vi "Msg.Event.Fire.vi"(8 "Error (in)":errorcluster, 9 "Data":variant, 10 "Message":string, 11 "Msg.Event.Ref":T1) -> (0 "Error (out)":errorcluster, 3 "Msg.Event.Ref (out)":T1)   [LabVIEW 2023]
doc: "Used to fire a user event."
uses:
  Msg.Event.Ref.ctl
  Msg.Data.ctl
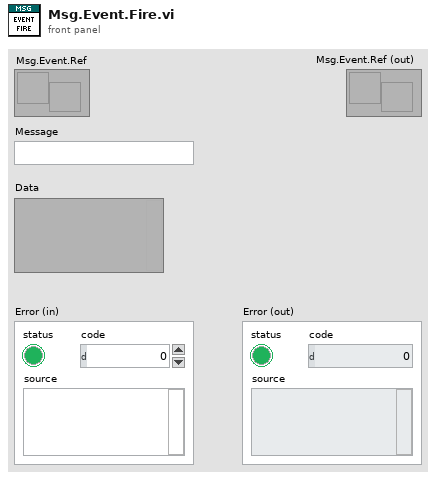
[diagram p1: front panel]
types:
  T1 = typedef "Msg.Event.Ref.ctl" = refnum<user-event>
  T2 = typedef "Msg.Data.ctl" = cluster{"Message":string, "Data":variant}
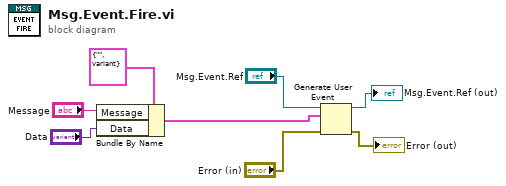
[diagram p0: block diagram]
diagram:
  n1 = Bundle By Name(cluster=T2 {"Message"="", "Data"=variant} ("Msg.Q.Data"), "Message"="Message", "Data"="Data") -> (w1:T2)
  n2 = Generate User Event(user event="Msg.Event.Ref", event data cluster=w1, error in="Error (in)") -> (user event out=→"Msg.Event.Ref (out)":T1, error out=→"Error (out)":errorcluster)  [unwired: 1 in]
